vi "Ruta.vi"() -> ()   [LabVIEW 2012]
uses:
  <vilib>/addons/database/Auxilliary.llb/DB Tools Cursor Type.ctl
  <vilib>/addons/database/Connection.llb/DB Tools Open Connec (Path).vi
  <vilib>/addons/database/Connection.llb/Conn Execute.vi
  <vilib>/addons/database/Recordset.llb/Rec Fetch String Data (R).vi
  <vilib>/addons/database/Recordset.llb/Rec Destroy - Connection.vi
  <vilib>/addons/database/Recordset.llb/Rec Get Recordset Properties (R).vi
  <vilib>/addons/database/NI_Database_API.lvlib
panel:
  in  "?":refnum<k7>(container)
  in  "Trazar":bool
  in  "FINAL":u16(ring) items=["-", "POC0", "POC1", "POC2", "POC3", "POC4", "POC5", "POC6", "POC7", "POC8", "POC9", "POC10", "POC11", "POC12", "POC13", "POC14", "POC15", "POC16", "POC17", "POC18", "POC19", "POC20", "POC21", "POC22", "POC23", "POC24", "POC25", "POC26", "POC27", "POC28", "POC29", "POC30", "POC31", "POC32", "POC33", "POC34", "POC35", "POC36", "POC37", "POC38", "POC39", "POC40", "POC41", "POC42", "POC43", "POC44", "POC45", "POC46", "POC47", "POC48", "POC49", "POC50", "POC51", "POC52", "POC53", "POC54", "POC55", "POC56", "POC57", "POC58", "POC59", "POC60", "POC61", "POC62", "POC63", "POC64", "POC65", "POC66", "POC67", "POC68", "POC69", "POC70", "POC71", "POC72", "POC73", "POC74", "POC75", "POC76", "POC77", "POC78", "POC79", "POC80", "POC81", "POC82", "POC83", "POC84", "POC85", "POC86", "POC87", "POC88", "POC89", "POC90", "POC91", "POC92", "POC93", "POC94", "POC95", "POC96", "POC97", "POC98", "POC99"]
  in  "INICIO":u16(ring) items=["-", "POC0", "POC1", "POC2", "POC3", "POC4", "POC5", "POC6", "POC7", "POC8", "POC9", "POC10", "POC11", "POC12", "POC13", "POC14", "POC15", "POC16", "POC17", "POC18", "POC19", "POC20", "POC21", "POC22", "POC23", "POC24", "POC25", "POC26", "POC27", "POC28", "POC29", "POC30", "POC31", "POC32", "POC33", "POC34", "POC35", "POC36", "POC37", "POC38", "POC39", "POC40", "POC41", "POC42", "POC43", "POC44", "POC45", "POC46", "POC47", "POC48", "POC49", "POC50", "POC51", "POC52", "POC53", "POC54", "POC55", "POC56", "POC57", "POC58", "POC59", "POC60", "POC61", "POC62", "POC63", "POC64", "POC65", "POC66", "POC67", "POC68", "POC69", "POC70", "POC71", "POC72", "POC73", "POC74", "POC75", "POC76", "POC77", "POC78", "POC79", "POC80", "POC81", "POC82", "POC83", "POC84", "POC85", "POC86", "POC87", "POC88", "POC89", "POC90", "POC91", "POC92", "POC93", "POC94", "POC95", "POC96", "POC97", "POC98", "POC99"]
  in  "stop":bool
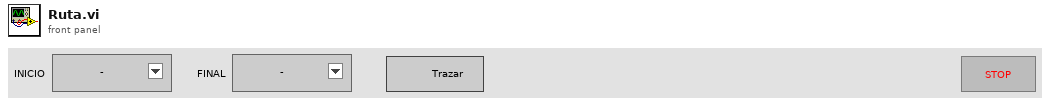
[diagram p1: front panel]
types:
  T1 = typedef "NI_Database_API.lvlib/Conn ObjectReference.ctl" = refnum<k1>
  T2 = enum16{"POC", "Imei", "Evento", "Lat", "Lon", "F_H_eve", "F_H_rec", "AVL_N", "AVL_pass", "Propietario", "Razon_Social", "Direccion", "Propietario_N", "Ciudad", "Marca", "Ruta", "N_Ruta", "Auditor", "Auditor_N"}
  T3 = typedef "NI_Database_API.lvlib/DB Tools Cursor Type.ctl" = enum16{"forward-only", "keyset", "dynamic", "static"}
  T4 = typedef "NI_Database_API.lvlib/Rec ObjectReference.ctl" = refnum<k1>
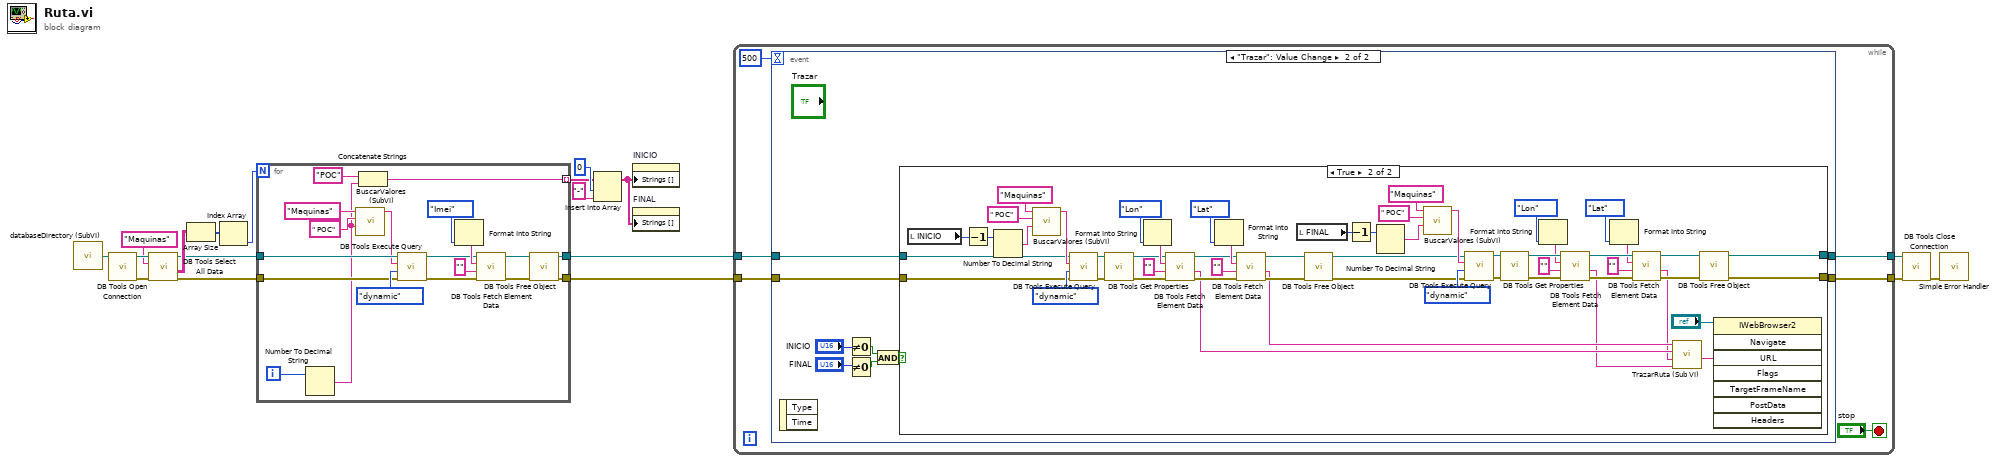
[diagram p0: block diagram]
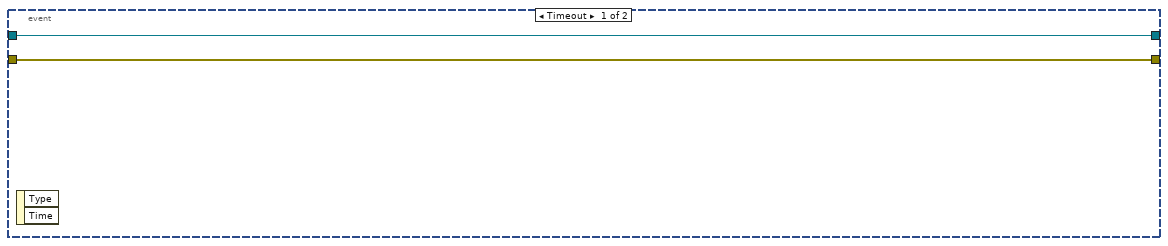
[diagram p2: hidden frame]
diagram:
  n1 = call "databaseDirectory (SubVI).vi"() -> ("Application Directory"=w6:path)  [unwired: 1 in]
  n2 = call-poly <vilib>:"DB Tools Open Connection.vi"("connection information"=w6) -> ("error out"=w11:errorcluster, "connection reference"=w10:T1)  [unwired: 7 in]
  n3 = call <vilib>:"DB Tools Select All Data.vi"("error in (no error)"=w11, "table"="Maquinas", "connection reference"=w10) -> ("error out"=w5:errorcluster, "data"=w13:string[][], "connection reference out"=w9:T1)  [unwired: 3 in]
  n4 = Array Size(array=w13) -> (size(s)=w12:i32[])
  n5 = Index Array(array=w12) -> (element=w7:i32)  [unwired: 1 in]
  n6 = for {
    N: w7 -> [_]
    tunnel: w9 -> [w32]
    tunnel: w5 -> [w33]
    tunnel: [w31] -> w3
    tunnel: [w30] -> w2
    tunnel: [w20] -> w4 mode=indexing
    i -> [w19]
    n7 = Number To Decimal String(number=w19) -> (decimal integer string=w22:string)  [unwired: 1 in]
    n8 = call "BuscarValores (SubVI).vi"("="=w22, "Columna"=" POC" ("Substring"), "Tabla"="Maquinas" ("table")) -> ("String"=w29:string)  [unwired: 8 in]
    n9 = Concatenate Strings("POC" ("string"), w22) -> (w20:string)
    n10 = call-poly <vilib>:"DB Tools Execute Query.vi"("error in (no error)"=w33, "cursor type"=DB_Tools_Cursor_Type."dynamic", "SQL query"=w29, "connection reference"=w32) -> ("error out"=w25:errorcluster, "recordset reference"=w26:T4)  [unwired: 4 in]
    n11 = Format Into String(T2."Imei") -> (resulting string=w37:string)  [unwired: 3 in, 1 out]
    n12 = call-poly <vilib>:"DB Tools Fetch Element Data.vi"("error in (no error)"=w25, "type"="", "column index"=w37, "recordset reference"=w26) -> ("error out"=w23:errorcluster, "recordset reference out"=w24:T4)  [unwired: 3 in, 1 out]
    n13 = call-poly <vilib>:"DB Tools Free Object.vi"("error in (no error)"=w23, "recordset reference"=w24) -> ("error out"=w30:errorcluster, "connection reference"=w31:T1)  [unwired: 8 in]
  }
  n14 = Insert Into Array(array=w4, index=0, new element="-" ("new element/subarray")) -> (w1:string[])
  n15 = property on="INICIO" class="Ring (strict)"("Strings []"=w1) -> ()  [unwired: 2 in, 2 out]
  n16 = property on="FINAL" class="Ring (strict)"("Strings []"=w1) -> ()  [unwired: 2 in, 2 out]
  n17 = while {
    tunnel: w3 -> [w43]
    tunnel: w2 -> [w42]
    tunnel: [w39] -> w17
    tunnel: [w38] -> w16
    stop <- "stop" stop-if-true
    n18 = event shown="[1] \"Trazar\": Value Change" {
      selector: _ -> [_ _]
      dyn-events: _ -> [_ _]
      timeout: 500 -> [_ _]
      tunnel: w43 -> [w45 w46]
      tunnel: w42 -> [w44 w47]
      tunnel: [w45 _] -> w39
      tunnel: [w44 _] -> w38
      event Timeout {
        n19 = event-data() -> ()  [unwired: 1 in, 2 out]
      }
      event "Trazar": Value Change {
        n20 = event-data() -> ()  [unwired: 1 in, 2 out]
        n21 = Not Equal To 0?(x="INICIO") -> (x != 0?=w51:bool)
        n22 = Not Equal To 0?(x="FINAL") -> (x != 0?=w52:bool)
        n23 = And(x=w51, y=w52) -> (x .and. y?=w50:bool)
        n24 = case shown="True" w50 {
          tunnel: [w54 w68] -> _
          tunnel: [w53 w67] -> _
          tunnel: w47 -> [w53 w62]
          tunnel: w46 -> [w54 w61]
          frame False {
          }
          frame True {
            n25 = local read "INICIO"() -> (w55:u16)
            n26 = Decrement(x=w55) -> (x-1=w56:u16)
            n27 = Number To Decimal String(number=w56) -> (decimal integer string=w70:string)  [unwired: 1 in]
            n28 = call "BuscarValores (SubVI).vi"("="=w70, "Columna"=" POC" ("Substring"), "Tabla"="Maquinas" ("table")) -> ("String"=w97:string)  [unwired: 8 in]
            n29 = call-poly <vilib>:"DB Tools Execute Query.vi"("error in (no error)"=w62, "cursor type"=DB_Tools_Cursor_Type."dynamic", "SQL query"=w97, "connection reference"=w61) -> ("error out"=w104:errorcluster, "recordset reference"=w105:T4)  [unwired: 4 in]
            n30 = call-poly <vilib>:"DB Tools Get Properties.vi"("error in (no error)"=w104, "recordset reference"=w105) -> ("error out"=w93:errorcluster, "recordset reference out"=w94:T4)  [unwired: 3 in, 1 out]
            n31 = Format Into String(T2."Lon") -> (resulting string=w108:string)  [unwired: 3 in, 1 out]
            n32 = call-poly <vilib>:"DB Tools Fetch Element Data.vi"("error in (no error)"=w93, "type"="", "column index"=w108, "recordset reference"=w94) -> ("error out"=w99:errorcluster, "data"=w65:string, "recordset reference out"=w100:T4)  [unwired: 3 in]
            n33 = Format Into String(T2."Lat") -> (resulting string=w101:string)  [unwired: 3 in, 1 out]
            n34 = call-poly <vilib>:"DB Tools Fetch Element Data.vi"("error in (no error)"=w99, "type"="", "column index"=w101, "recordset reference"=w100) -> ("error out"=w91:errorcluster, "data"=w66:string, "recordset reference out"=w92:T4)  [unwired: 3 in]
            n35 = local read "FINAL"() -> (w57:u16)
            n36 = call-poly <vilib>:"DB Tools Free Object.vi"("error in (no error)"=w91, "recordset reference"=w92) -> ("error out"=w71:errorcluster, "connection reference"=w72:T1)  [unwired: 8 in]
            n37 = Decrement(x=w57) -> (x-1=w58:u16)
            n38 = Number To Decimal String(number=w58) -> (decimal integer string=w69:string)  [unwired: 1 in]
            n39 = call "BuscarValores (SubVI).vi"("="=w69, "Columna"=" POC" ("Substring"), "Tabla"="Maquinas" ("table")) -> ("String"=w84:string)  [unwired: 8 in]
            n40 = call-poly <vilib>:"DB Tools Execute Query.vi"("error in (no error)"=w71, "cursor type"=DB_Tools_Cursor_Type."dynamic", "SQL query"=w84, "connection reference"=w72) -> ("error out"=w77:errorcluster, "recordset reference"=w76:T4)  [unwired: 4 in]
            n41 = call-poly <vilib>:"DB Tools Get Properties.vi"("error in (no error)"=w77, "recordset reference"=w76) -> ("error out"=w88:errorcluster, "recordset reference out"=w87:T4)  [unwired: 3 in, 1 out]
            n42 = Format Into String(T2."Lon") -> (resulting string=w73:string)  [unwired: 3 in, 1 out]
            n43 = call-poly <vilib>:"DB Tools Fetch Element Data.vi"("error in (no error)"=w88, "type"="", "column index"=w73, "recordset reference"=w87) -> ("error out"=w82:errorcluster, "data"=w64:string, "recordset reference out"=w81:T4)  [unwired: 3 in]
            n44 = Format Into String(T2."Lat") -> (resulting string=w80:string)  [unwired: 3 in, 1 out]
            n45 = call-poly <vilib>:"DB Tools Fetch Element Data.vi"("error in (no error)"=w82, "type"="", "column index"=w80, "recordset reference"=w81) -> ("error out"=w90:errorcluster, "data"=w63:string, "recordset reference out"=w89:T4)  [unwired: 3 in]
            n46 = call "TrazarRuta (Sub VI).vi"("LAT INI"=w66, "LNG INI"=w65, "LAT END"=w63, "LNG END"=w64) -> ("URL"=w59:string)  [unwired: 1 in]
            n47 = call-poly <vilib>:"DB Tools Free Object.vi"("error in (no error)"=w90, "recordset reference"=w89) -> ("error out"=w67:errorcluster, "connection reference"=w68:T1)  [unwired: 8 in]
            n48 = invoke class="IWebBrowser2" method="Navigate"(reference="?", "URL"=w59) -> ()  [unwired: 6 in, 8 out]
          }
        }
      }
    }
  }
  n49 = call <vilib>:"DB Tools Close Connection.vi"("error in (no error)"=w16, "connection reference"=w17) -> ("error out"=w18:errorcluster)  [unwired: 5 in]
  n50 = call <vilib>:"Simple Error Handler.vi"("error in (no error)"=w18) -> ()  [unwired: 4 in, 5 out]
